vi "dfd_DFXPSimu Casting (scaler)64bits.vi"(5 "quantize output?(T)":bool=TRUE, 7 "op params":T2={"source"=0, "is floating?"=FALSE, "o-mode"=enum."Wrap", "q-mode"=enum."Nearest", "wl"=0, "high limit"=0, "low limit"=0, "iwl"=0, "sign?"=TRUE} {"source" items=["Coef a/k"=0, "Coef b/v"=7, "Input"=1, "Output"=2, "Multiplicand"=3, "Product"=4, "Sum"=5, "Delay"=6, "Gain"=8]}, 8 "filtering statistics in":T6(array[cluster]) {"statistics information"."min value" format="%.2f"; "statistics information"."max value" format="%.2f"; "Quantizer Source" items=["Coefficients a/k"=0, "Coefficients b/v"=7, "Input"=1, "Output"=2, "Multiplicand"=3, "Product"=4, "Sum"=5, "Delay"=6]}, 11 "Value in":T1={"value"=0, "wl"=0, "iwl"=0, "Signed"=TRUE} {"value" format="%.0x"}) -> (0 "filtering statistics out":T6(array[cluster]) {"statistics information"."min value" format="%.2f"; "statistics information"."max value" format="%.2f"; "Quantizer Source" items=["Coefficients a/k"=0, "Coefficients b/v"=7, "Input"=1, "Output"=2, "Multiplicand"=3, "Product"=4, "Sum"=5, "Delay"=6]}, 3 "Value out":T1={"value"=0, "wl"=0, "iwl"=0, "Signed"=TRUE} {"value" format="%.0x"})   [LabVIEW 2017, in "NI_DigFilter_FXP.lvlib"]
uses:
  <vilib>/addons/Digital Filter Design/NI_DigFilter_FXP.lvlib
  <vilib>/addons/Digital Filter Design/_Objects.llb/dfd_DFXP Data Type (scaler).ctl
  <vilib>/addons/Digital Filter Design/_Objects.llb/DFD Quantization Sources.ctl
  <vilib>/addons/Digital Filter Design/_Objects.llb/DFD FXP Statistics Data.ctl
  <vilib>/addons/Digital Filter Design/_Objects.llb/dfd_DFXP Operation Parameter.ctl
  <vilib>/addons/Digital Filter Design/_Objects.llb/dfd_Internal Quantization Srcs.ctl
  <vilib>/addons/Digital Filter Design/NI_DigFilterLicensed.lvlib
panel:
  in  "Value out type":T1={"value"=0, "wl"=0, "iwl"=0, "Signed"=TRUE} {"value" format="%.0x"}
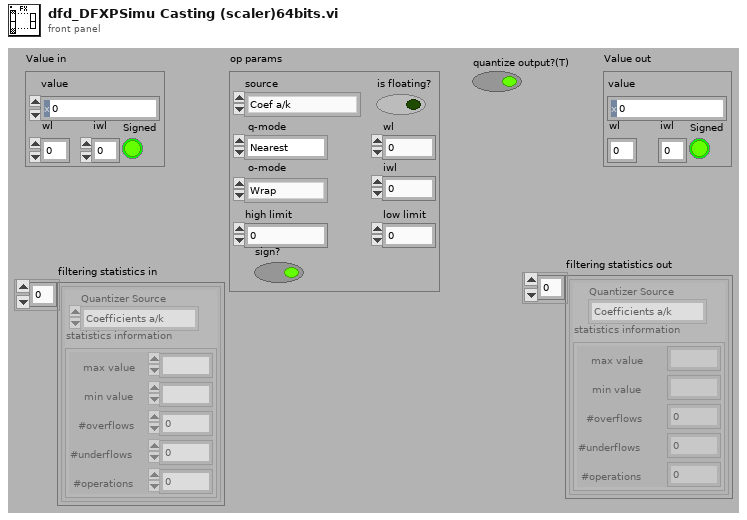
[diagram p1: front panel]
types:
  T1 = typedef "dfd_DFXP Data Type (scaler).ctl" = cluster{"value":i64, "wl":i16, "iwl":i16, "Signed":bool}
  T2 = typedef "dfd_DFXP Operation Parameter.ctl" = cluster{"source":T3, "is floating?":bool, "o-mode":enum16{"Saturation", "Wrap"}, "q-mode":enum16{"Nearest", "Truncation"}, "wl":i16, "high limit":i64, "low limit":i64, "iwl":i16, "sign?":bool}
  T3 = typedef "NI_DigFilterLicensed.lvlib/dfd_Internal Quantization Srcs.ctl" = u16
  T4 = typedef "NI_DigFilterLicensed.lvlib/DFD Quantization Sources.ctl" = u16
  T5 = typedef "NI_DigFilterLicensed.lvlib/DFD FXP Statistics Data.ctl" = cluster{"max value":ext, "min value":ext, "#overflows":i32, "#underflows":i32, "#operations":i32}
  T6 = cluster{"Quantizer Source":T4, "statistics information":T5}[]
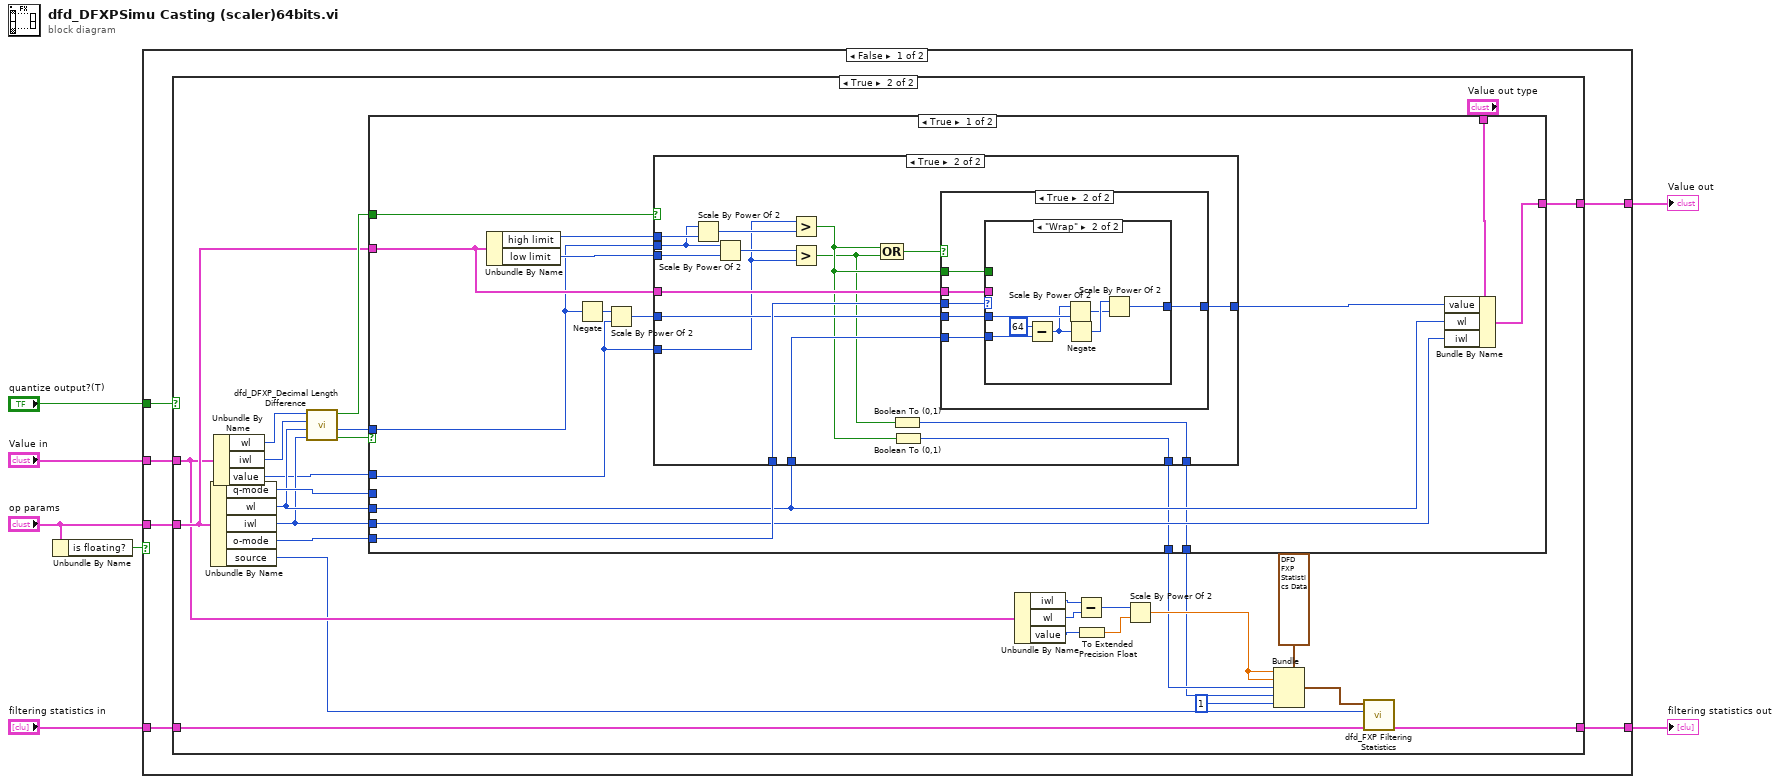
[diagram p0: block diagram]
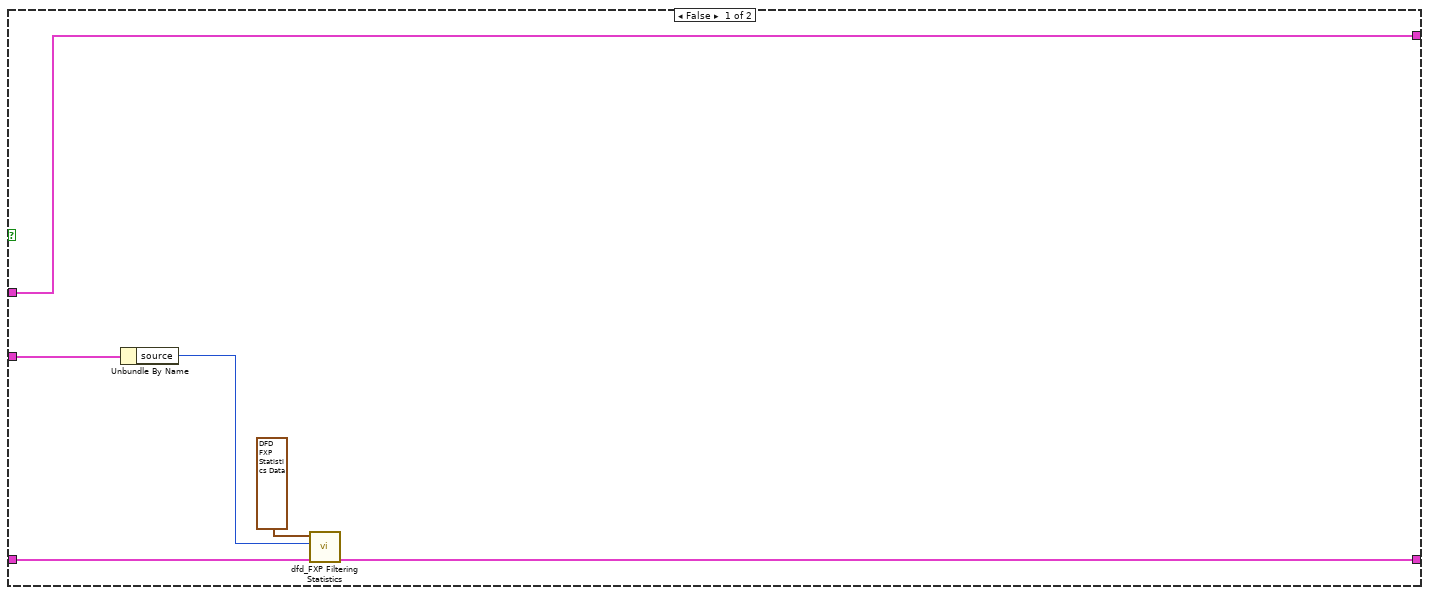
[diagram p2: hidden frame]
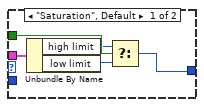
[diagram p5: hidden frame]
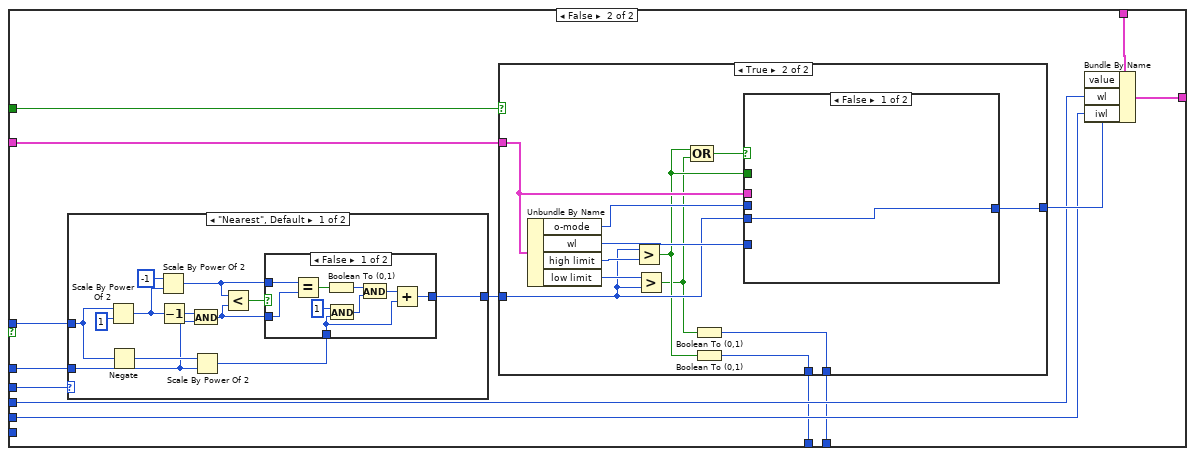
[diagram p6: hidden frame]
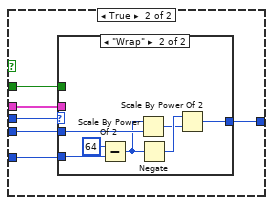
[diagram p8: hidden frame]
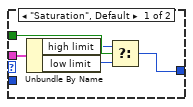
[diagram p9: hidden frame]
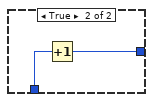
[diagram p10: hidden frame]
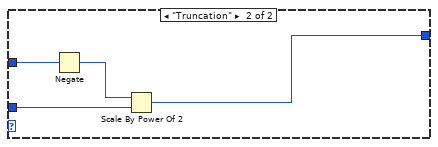
[diagram p11: hidden frame]
diagram:
  n1 = Unbundle By Name("op params") -> ("is floating?"=w1:bool)
  n2 = case shown="False" w1 {
    tunnel: [w13 w173] -> w7
    tunnel: [w12 w172] -> w6
    tunnel: "filtering statistics in" -> [w11 w172]
    tunnel: "Value in" -> [w10 w173]
    tunnel: "quantize output?(T)" -> [w9 _]
    tunnel: "op params" -> [w8 _]
    frame False {
      n3 = case shown="True" w9 {
        tunnel: [w18 w36] -> w13
        tunnel: w8 -> [w19 w39]
        tunnel: w10 -> [w18 w34]
        tunnel: w11 -> [w15 w33]
        tunnel: [w14 w21] -> w12
        frame False {
          n4 = Unbundle By Name(w19) -> ("source"=w17:T3)
          n5 = call <vilib>:"dfd_FXP Filtering Statistics.vi"("filtering statistics in"=w15, "source"=w17, "new data"=T5 {"max value"=-inf, "min value"=inf, "#overflows"=0, "#underflows"=0, "#operations"=1}) -> ("filtering statistics out"=w14:T6)  [unwired: 8 in]
        }
        frame True {
          n6 = Unbundle By Name(w39) -> ("q-mode"=w47:enum16{"Nearest", "Truncation"}, "wl"=w40:i16, "iwl"=w38:i16, "o-mode"=w41:enum16{"Saturation", "Wrap"}, "source"=w32:T3)
          n7 = Unbundle By Name(w34) -> ("wl"=w45:i16, "iwl"=w46:i16, "value"=w35:i64)
          n8 = call <vilib>:"dfd_DFXP_Decimal Length Difference.vi"("iwl 2"=w38, "wl 2"=w40, "iwl 1"=w46, "wl 1"=w45) -> ("fwl_diff <= 0?"=w44:bool, "fwl_diff"=w42:i16, "iwl_diff >= 0?"=w43:bool)  [unwired: 5 out]
          n9 = case shown="True" w44 {
            tunnel: w47 -> [_ w112]
            tunnel: w35 -> [w51 w111]
            tunnel: w39 -> [w60 w107]
            tunnel: w43 -> [w52 w109]
            tunnel: w42 -> [w50 w108]
            tunnel: w41 -> [w59 _]
            tunnel: w40 -> [w55 w104]
            tunnel: [w53 w102] -> w36
            tunnel: w38 -> [w54 w103]
            tunnel: "Value out type" -> [w57 w106]
            tunnel: [w49 w101] -> w24
            tunnel: [w48 w100] -> w23
            frame True {
              n10 = Unbundle By Name(w60) -> ("high limit"=w62:i64, "low limit"=w61:i64)
              n11 = Negate(x=w50) -> (-x=w63:i16)
              n12 = Scale By Power Of 2(n=w63, x=w51) -> (x*2^n=w58:i64)
              n13 = case shown="True" w52 {
                tunnel: w62 -> [_ w80]
                tunnel: w61 -> [_ w79]
                tunnel: w60 -> [_ w75]
                tunnel: w59 -> [_ w74]
                tunnel: w58 -> [w64 w73]
                tunnel: [w64 w65] -> w56
                tunnel: w55 -> [_ w72]
                tunnel: w51 -> [_ w71]
                tunnel: w50 -> [_ w70]
                tunnel: [_ w66] -> w49
                tunnel: [_ w67] -> w48
                frame False {
                }
                frame True {
                  n14 = Scale By Power Of 2(n=w70, x=w80) -> (x*2^n=w78:i64)
                  n15 = Scale By Power Of 2(n=w70, x=w79) -> (x*2^n=w77:i64)
                  n16 = Greater?(x=w71, y=w78) -> (0:w69:bool)
                  n17 = Greater?(x=w77, y=w71) -> (0:w68:bool)
                  n18 = Compound Arithmetic op=OR(w69, w68) -> (w76:bool)
                  n19 = Boolean To (0,1)(Boolean=w68) -> (0, 1=w67:i16)
                  n20 = Boolean To (0,1)(Boolean=w69) -> (0, 1=w66:i16)
                  n21 = case shown="True" w76 {
                    tunnel: w74 -> [_ w87]
                    tunnel: w69 -> [_ w86]
                    tunnel: [w81 w85] -> w65
                    tunnel: w72 -> [_ w84]
                    tunnel: w73 -> [w81 w83]
                    tunnel: w75 -> [_ w82]
                    frame False {
                    }
                    frame True {
                      n22 = case shown="\"Wrap\"" w87 {
                        tunnel: w86 -> [w91 _]
                        tunnel: [w88 w98] -> w85
                        tunnel: w84 -> [_ w99]
                        tunnel: w83 -> [_ w97]
                        tunnel: w82 -> [w92 _]
                        frame "Saturation", Default {
                          n23 = Unbundle By Name(w92) -> ("high limit"=w90:i64, "low limit"=w89:i64)
                          n24 = Select(t=w90, s=w91, f=w89) -> (s? t:f=w88:i64)
                        }
                        frame "Wrap" {
                          n25 = Subtract(x=i16 64, y=w99) -> (x-y=w95:i16)
                          n26 = Scale By Power Of 2(n=w95, x=w97) -> (x*2^n=w93:i64)
                          n27 = Negate(x=w95) -> (-x=w94:i16)
                          n28 = Scale By Power Of 2(n=w94, x=w93) -> (x*2^n=w98:i64)
                        }
                      }
                    }
                  }
                }
              }
              n29 = Bundle By Name(cluster=w57, "value"=w56, "wl"=w55, "iwl"=w54) -> (w53:T1)
            }
            frame False {
              n30 = case shown="\"Nearest\", Default" w112 {
                tunnel: w108 -> [w150 w171]
                tunnel: w111 -> [w153 w168]
                tunnel: [w146 w169] -> w110
                frame "Nearest", Default {
                  n31 = Scale By Power Of 2(n=w150, x=i64 1) -> (x*2^n=w151:i64)
                  n32 = Negate(x=w150) -> (-x=w156:i16)
                  n33 = Scale By Power Of 2(n=-1, x=w151) -> (x*2^n=w149:i64)
                  n34 = Decrement(x=w151) -> (x-1=w154:i64)
                  n35 = And(x=w154, y=w153) -> (x .and. y?=w148:i64)
                  n36 = Scale By Power Of 2(n=w156, x=w153) -> (x*2^n=w147:i64)
                  n37 = Less?(x=w149, y=w148) -> (x < y?=w145:bool)
                  n38 = case shown="False" w145 {
                    tunnel: w149 -> [w165 _]
                    tunnel: w148 -> [w164 _]
                    tunnel: w147 -> [w157 w167]
                    tunnel: [w158 w166] -> w146
                    frame False {
                      n39 = Equal?(x=w165, y=w164) -> (x = y?=w162:bool)
                      n40 = Boolean To (0,1)(Boolean=w162) -> (0, 1=w161:i16)
                      n41 = And(x=i64 1, y=w157) -> (x .and. y?=w160:i64)
                      n42 = And(x=w161, y=w160) -> (x .and. y?=w159:i64)
                      n43 = Add(x=w159, y=w157) -> (x+y=w158:i64)
                    }
                    frame True {
                      n44 = Increment(x=w167) -> (x+1=w166:i64)
                    }
                  }
                }
                frame "Truncation" {
                  n45 = Negate(x=w171) -> (-x=w170:i16)
                  n46 = Scale By Power Of 2(n=w170, x=w168) -> (x*2^n=w169:i64)
                }
              }
              n47 = case shown="True" w109 {
                tunnel: w110 -> [w113 w120]
                tunnel: w107 -> [_ w119]
                tunnel: [w113 w118] -> w105
                tunnel: [_ w115] -> w101
                tunnel: [_ w114] -> w100
                frame False {
                }
                frame True {
                  n48 = Unbundle By Name(w119) -> ("o-mode"=w122:enum16{"Saturation", "Wrap"}, "wl"=w121:i16, "high limit"=w125:i64, "low limit"=w124:i64)
                  n49 = Greater?(x=w120, y=w125) -> (0:w117:bool)
                  n50 = Greater?(x=w124, y=w120) -> (0:w116:bool)
                  n51 = Compound Arithmetic op=OR(w117, w116) -> (w123:bool)
                  n52 = Boolean To (0,1)(Boolean=w116) -> (0, 1=w114:i16)
                  n53 = Boolean To (0,1)(Boolean=w117) -> (0, 1=w115:i16)
                  n54 = case shown="False" w123 {
                    tunnel: w122 -> [_ w132]
                    tunnel: w117 -> [_ w131]
                    tunnel: [w126 w130] -> w118
                    tunnel: w121 -> [_ w129]
                    tunnel: w120 -> [w126 w128]
                    tunnel: w119 -> [_ w127]
                    frame False {
                    }
                    frame True {
                      n55 = case shown="\"Wrap\"" w132 {
                        tunnel: w131 -> [w136 _]
                        tunnel: [w133 w143] -> w130
                        tunnel: w129 -> [_ w144]
                        tunnel: w128 -> [_ w142]
                        tunnel: w127 -> [w137 _]
                        frame "Saturation", Default {
                          n56 = Unbundle By Name(w137) -> ("high limit"=w135:i64, "low limit"=w134:i64)
                          n57 = Select(t=w135, s=w136, f=w134) -> (s? t:f=w133:i64)
                        }
                        frame "Wrap" {
                          n58 = Subtract(x=i16 64, y=w144) -> (x-y=w140:i16)
                          n59 = Scale By Power Of 2(n=w140, x=w142) -> (x*2^n=w138:i64)
                          n60 = Negate(x=w140) -> (-x=w139:i16)
                          n61 = Scale By Power Of 2(n=w139, x=w138) -> (x*2^n=w143:i64)
                        }
                      }
                    }
                  }
                }
              }
              n62 = Bundle By Name(cluster=w106, "value"=w105, "wl"=w104, "iwl"=w103) -> (w102:T1)
            }
          }
          n63 = Unbundle By Name(w34) -> ("iwl"=w31:i16, "wl"=w30:i16, "value"=w28:i64)
          n64 = Subtract(x=w31, y=w30) -> (x-y=w29:i16)
          n65 = To Extended Precision Float(1:w28) -> (0:w27:ext)
          n66 = Scale By Power Of 2(n=w29, x=w27) -> (x*2^n=w25:ext)
          n67 = Bundle(cluster=T5 {"max value"=-inf, "min value"=inf, "#overflows"=0, "#underflows"=0, "#operations"=1} ("new data"), "max value"=w25, "min value"=w25, "#overflows"=w24, "#underflows"=w23, "#operations"=1) -> (w20:T5)
          n68 = call <vilib>:"dfd_FXP Filtering Statistics.vi"("filtering statistics in"=w33, "source"=w32, "new data"=w20) -> ("filtering statistics out"=w21:T6)  [unwired: 8 in]
        }
      }
    }
    frame True {
    }
  }
  "Value out" <- w7
  "filtering statistics out" <- w6
